vi "Volt_AutoScalling_Osc_Dual_Channel_Control.vi"(0 "VISA Oscilloscope":refnum<visa-resource-name>, 5 "Voltage In":dbl, 7 "N Channels":dbl, 9 "Offset Divider":dbl=8.0, 11 "error in":errorcluster) -> (4 "VISA resource name out":refnum<visa-resource-name>, 15 "error out":errorcluster)   [LabVIEW 2009]
uses:
  Sum_Abrilader/L0_Sum_Adder Folder/C/Program Files/National Instruments/LabVIEW 2012/instr.lib/Agilent 8000 Series/Agilent 8000 Series.lvlib
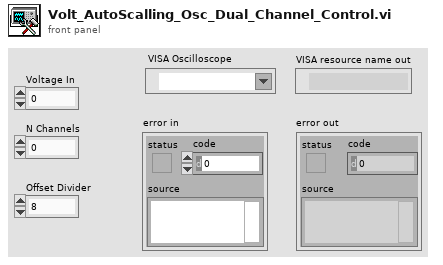
[diagram p1: front panel]
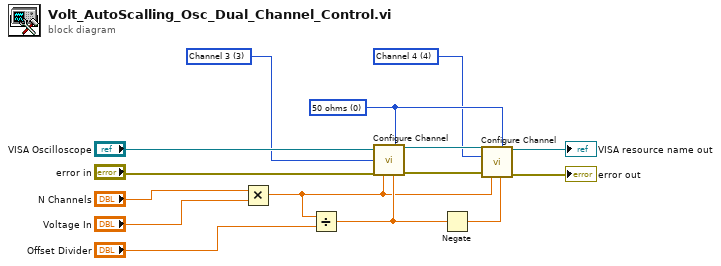
[diagram p0: block diagram]
diagram:
  w4 = 3 items=["Channel 1"=1, "Channel 2"=2, "Channel 3"=3, "Channel 4"=4] ("Channel (1: Channel 1)")
  w14 = u32 0 items=["50 ohms", "1 Mohms"] ("Input Impedance (1: 1 Mohms)")
  w13 = 4 items=["Channel 1"=1, "Channel 2"=2, "Channel 3"=3, "Channel 4"=4] ("Channel (1: Channel 1)")
  n1 = Multiply(x="N Channels", y="Voltage In") -> (x*y=w10:dbl)
  n2 = Divide(x=w10, y="Offset Divider") -> (x/y=w11:dbl)
  n3 = call "Configure Channel.vi"("VISA resource name"="VISA Oscilloscope", "Input Impedance (1: 1 Mohms)"=w14, "Channel (1: Channel 1)"=w4, "error in (no error)"="error in", "Vertical Range (2.0 V)"=w10, "Vertical Offset (0.0 V)"=w11) -> ("VISA resource name out"=w15:refnum<visa-resource-name>, "error out"=w5:errorcluster)  [unwired: 8 in]
  n4 = Negate(x=w11) -> (-x=w12:dbl)
  n5 = call "Configure Channel.vi"("VISA resource name"=w15, "Input Impedance (1: 1 Mohms)"=w14, "Channel (1: Channel 1)"=w13, "error in (no error)"=w5, "Vertical Range (2.0 V)"=w10, "Vertical Offset (0.0 V)"=w12) -> ("VISA resource name out"=→"VISA resource name out":refnum<visa-resource-name>, "error out"=→"error out":errorcluster)  [unwired: 8 in]
